vi "OE1201_Configure Ref Phase.vi"(7 "OE1201_Configure Ref Phase":T1={"Internal Frequency(Hz)"=1000.0, "External Ref Trigger"=0, "Reference Source"=0, "Phase  (degree)"=0.0} {"Phase  (degree)" format="%#.2g"; "Reference Source" items=["External", "Internal"]; "External Ref Trigger" items=["TTL Rising Edge", "Sine Zero Crossing"]; "Internal Frequency(Hz)" min=0.001 max=120000.0 format="%#_10g"}, 8 "Error in (no error)":errorcluster caption="error out（no error）", 9 "Remote Mode":u16(ring) items=["USB", "RS232"], 11 "VISA resource name":refnum<visa-resource-name>) -> (0 "Error out":errorcluster caption="error out", 1 "Output String":string, 3 "VISA resource  out":refnum<visa-resource-name>)   [LabVIEW 2011]
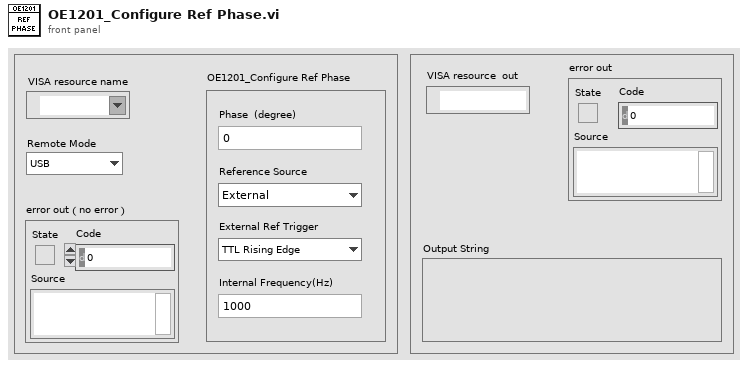
[diagram p1: front panel]
types:
  T1 = cluster{"Internal Frequency(Hz)":dbl, "External Ref Trigger":u16, "Reference Source":u16, "Phase  (degree)":dbl}
  T2 = enum16{"ISRC", "IGND", "ICPL", "ILIN", "PHAS", "FMOD", "RSLP", "FREQ", "SWPT", "SLLM", "SULM", "SSLL", "SSLG", "STLM", "SWRM", "IRNG", "SENS", "RMOD", "OFLT", "OFSL", "SYNC", "DMOD", "HARM", "DARB", "SWVT", "SLVL", "SVLL", "SVUL", "SVSL", "SVSG", "SVTM", "SVRM", "RALL", "SNAP", "OUTP", "OAUX", "COUT", "CAUX", "COFP", "CEXP", "FPOP", "OEXP", "*IDN", "*RST", "OVLD", "INOV", "GNOV", "*PLL", "SSET", "RSET", "AGAN", "APHS", "ARSV", "ASCL", "EQCD", "EQCS", "SPED", "SRAT", "SLEN", "SSLE", "STRG", "SPRM", "STRD", "PAUS", "REST", "SPTS", "TRCA", "TEMP", "RSTU", "IHNZ", "DEQU", "SADD", "ARNG", "CSPE", "ISRCD", "IGNDD", "ICPLD", "ILIND", "PHASD", "FMODD", "RSLPD", "FREQD", "SWPTD", "SLLMD", "SULMD", "SSLLD", "SSLGD", "STLMD", "SWRMD", "SENSD", "RMODD", "OFLTD", "OFSLD", "SYNCD", "HARMD", "EQCDD", "EQCSD", "SNAPD", "OUTPD", "SWVTD", "SLVLD", "SVLLD", "SVULD", "SVSLD", "SVSGD", "SVTMD", "SVRMD", "SVDCD", "ARSVD", "AGAND", "APHSD", "ASCLD", "FPOPD", "CAUXD", "OEXPD", "SPEDD", "SRATD", "SLEND", "SSLED", "STRGD", "SPRMD", "STRDD", "PAUSD", "RESTD", "SPTSD", "TRCAD", "*IDND", "*RSTD", "INOVD", "GNOVD", "*PLLD", "SSETD", "RSETD"}
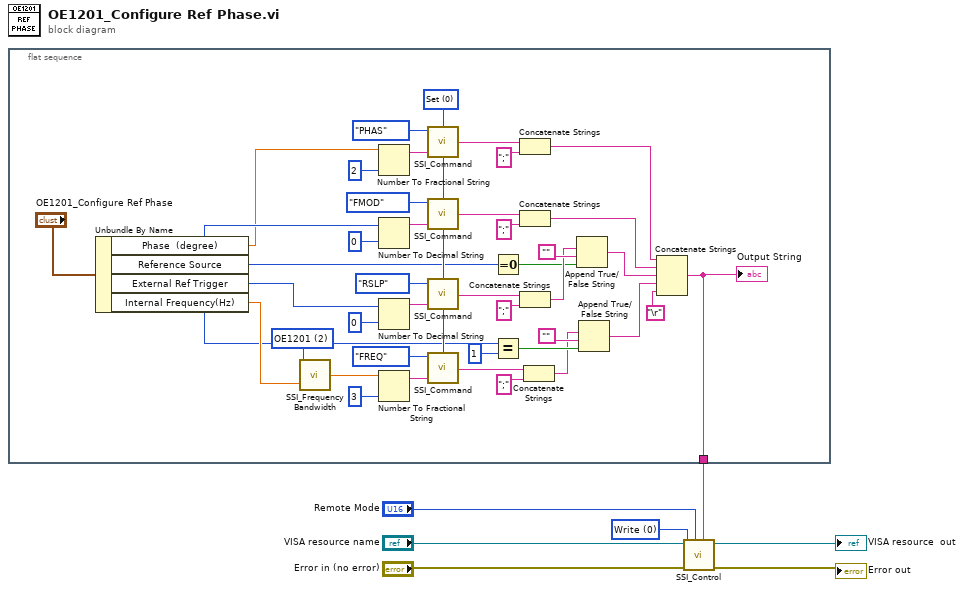
[diagram p0: block diagram]
diagram:
  w6 = u16 0 items=["Write", "Read"] ("Control")
  n1 = flat-sequence {
    tunnel: [w11] -> w1
    frame #0 {
      w34 = u16 0 items=["Set", "Query"] ("Opera")
      w35 = u16 2 items=["OE1022", "OE1022D", "OE1201", "OE1311", "OE1351", "OE1301", "OE2031-10M", "OE2041-30M", "OE2041-60M"] ("Instrument Mode")
      n2 = Unbundle By Name("OE1201_Configure Ref Phase") -> ("Phase  (degree)"=w8:dbl, "Reference Source"=w12:u16, "External Ref Trigger"=w13:u16, "Internal Frequency(Hz)"=w14:dbl)
      n3 = call "SSI_Frequency Bandwidth.vi"("Frequency"=w14, "Instrument Mode"=w35) -> ("Output"=w36:dbl)  [unwired: 1 in]
      n4 = Number To Fractional String(number=w8, precision (6)=i16 2 ("精度(6)")) -> (F-format string=w47:string)  [unwired: 2 in]
      n5 = Number To Decimal String(number=w12, width (-)=i16 0 ("精度(6)")) -> (decimal integer string=w44:string)
      n6 = Number To Decimal String(number=w13, width (-)=i16 0 ("精度(6)")) -> (decimal integer string=w41:string)
      n7 = Number To Fractional String(number=w36, precision (6)=i16 3 ("精度(6)")) -> (F-format string=w38:string)  [unwired: 2 in]
      n8 = call "SSI_Command.vi"("Opera"=w34, "Paramter"=w47, "Command Type"=T2."PHAS") -> ("Output string"=w24:string)  [unwired: 1 in]
      n9 = call "SSI_Command.vi"("Opera"=w34, "Paramter"=w44, "Command Type"=T2."FMOD") -> ("Output string"=w29:string)  [unwired: 1 in]
      n10 = call "SSI_Command.vi"("Opera"=w34, "Paramter"=w41, "Command Type"=T2."RSLP") -> ("Output string"=w22:string)  [unwired: 1 in]
      n11 = call "SSI_Command.vi"("Opera"=w34, "Paramter"=w38, "Command Type"=T2."FREQ") -> ("Output string"=w27:string)  [unwired: 1 in]
      n12 = Equal To 0?(x=w12) -> (x = 0?=w16:bool)
      n13 = Equal?(x=w12, y=u16 1) -> (x = y?=w32:bool)
      n14 = Concatenate Strings(w24, ";" ("替换字符串(\"\")")) -> (w21:string)
      n15 = Concatenate Strings(w29, ";" ("替换字符串(\"\")")) -> (w19:string)
      n16 = Concatenate Strings(w22, ";" ("替换字符串(\"\")")) -> (w17:string)
      n17 = Concatenate Strings(w27, ";" ("替换字符串(\"\")")) -> (w26:string)
      n18 = Append True/False String(1:w16, 2:"", 3:w17) -> (0:w15:string)  [unwired: 1 in]
      n19 = Append True/False String(1:w32, 2:"", 3:w26) -> (0:w20:string)  [unwired: 1 in]
      n20 = Concatenate Strings(w21, w19, w15, w20, "\r") -> (w11:string)
      "Output String" <- w11
    }
  }
  n21 = call "SSI_Control.vi"("Write Buffer"=w1, "Remote Mode"="Remote Mode", "Error in (no error)"="Error in (no error)", "Control"=w6, "VISA resource name"="VISA resource name") -> ("Error out"=→"Error out":errorcluster, "VISA resource  out"=→"VISA resource  out":refnum<visa-resource-name>)  [unwired: 3 in, 2 out]
